vi "ep_Kaiser Parameters.vi"(6 "fs [Hz]":dbl=1.0 format="%.2f", 8 "error in (no error)":errorcluster, 9 "A stop [dB]":dbl=72.0 format="%.2f", 11 "delta f [Hz]":dbl=0.1 format="%.2f") -> (0 "error out":errorcluster, 1 "beta":dbl format="%.2f", 3 "order":i32)   [LabVIEW 2012, in "NI_EP_Resample_Host.lvlib"]
uses:
  <vilib>/addons/Electrical Power/PQ/Resampling/NI_EP_Resample_Host.lvlib
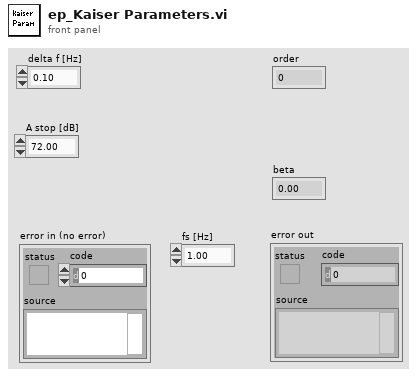
[diagram p1: front panel]
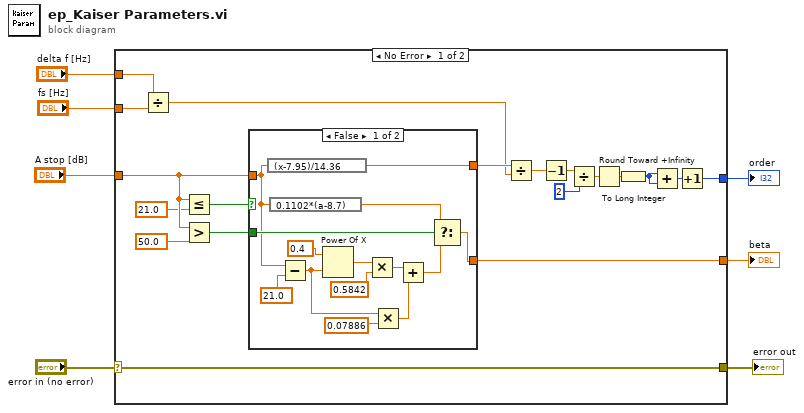
[diagram p0: block diagram]
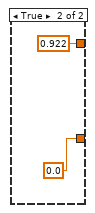
[diagram p2: hidden frame]
diagram:
  n1 = case shown="No Error" "error in (no error)" {
    selector: "error in (no error)" -> [w16 w43]
    tunnel: [w26 _] -> w7
    tunnel: "A stop [dB]" -> [w25 _]
    tunnel: "fs [Hz]" -> [w20 _]
    tunnel: "delta f [Hz]" -> [w19 _]
    tunnel: [w8 _] -> w3
    tunnel: [w16 w43] -> w1
    frame No Error {
      n2 = Divide(x=w19, y=w20) -> (x/y=w17:dbl)
      n3 = Less Or Equal?(x=w25, y=21.0) -> (x <= y?=w23:bool)
      n4 = Greater?(x=w25, y=50.0) -> (0:w24:bool)
      n5 = case shown="False" w23 {
        tunnel: [w39 0.0] -> w26
        tunnel: [w40 0.922] -> w18
        tunnel: w24 -> [w38 _]
        tunnel: w25 -> [w36 _]
        frame False {
          n6 = expression code="(x-7.95)/14.36"(w36) -> (w40:dbl)
          n7 = expression code="0.1102*(a-8.7)"(w36) -> (w37:dbl)
          n8 = Subtract(x=w36, y=21.0) -> (x-y=w30:dbl)
          n9 = Power Of X(1:w30, 2:0.4 ("y")) -> (0:w33:dbl)
          n10 = Multiply(x=w33, y=0.5842) -> (x*y=w29:dbl)
          n11 = Multiply(x=w30, y=0.07886) -> (x*y=w28:dbl)
          n12 = Add(x=w29, y=w28) -> (x+y=w27:dbl)
          n13 = Select(t=w37, s=w38, f=w27) -> (s? t:f=w39:dbl)
        }
        frame True {
        }
      }
      n14 = Divide(x=w18, y=w17) -> (x/y=w9:dbl)
      n15 = Decrement(x=w9) -> (x-1=w10:dbl)
      n16 = Divide(x=w10, y=2) -> (x/y=w13:dbl)
      n17 = Round Toward +Infinity(x=w13) -> (ceil(x): smallest int >= x=w14:dbl)
      n18 = To Long Integer(number=w14) -> (32bit integer=w11:i32)
      n19 = Add(x=w11, y=w11) -> (x+y=w12:i32)
      n20 = Increment(x=w12) -> (x+1=w8:i32)
    }
    frame Error {
    }
  }
  "order" <- w3
  "beta" <- w7
  "error out" <- w1
